vi "Read XML Parameters File_Parse Read Data_Convert sdi element.vi"(8 "error in (no error)":errorcluster, 11 "sdi":i32(ring) items=["All", "Item00", "Item01", "Item10", "Item11"]) -> (0 "error out":errorcluster, 2 "SDIValue":u8, 3 "SDI_Enabled":bool)   [LabVIEW 2019]
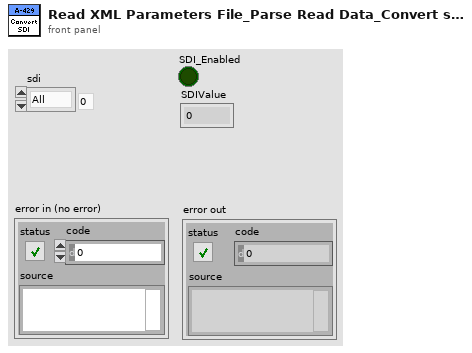
[diagram p1: front panel]
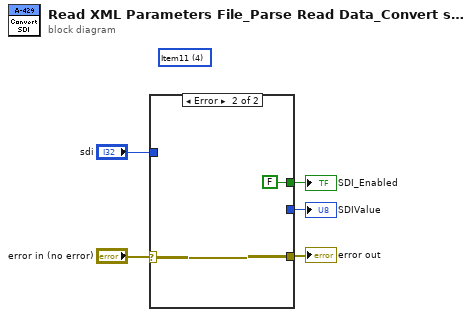
[diagram p0: block diagram]
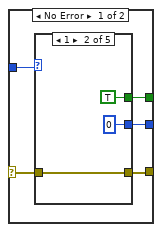
[diagram p2: hidden frame]
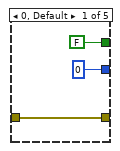
[diagram p3: hidden frame]
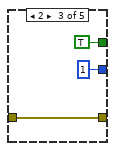
[diagram p4: hidden frame]
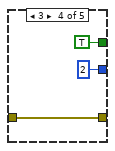
[diagram p5: hidden frame]
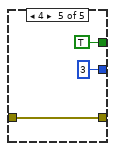
[diagram p6: hidden frame]
diagram:
  (unwired) 4 items=["All", "Item00", "Item01", "Item10", "Item11"] ("sdi")
  n1 = case shown="Error" "error in (no error)" {
    selector: "error in (no error)" -> [w9 w27]
    tunnel: [w8 w27] -> w4
    tunnel: "sdi" -> [w10 _]
    tunnel: [w7 FALSE] -> w2
    tunnel: [w6 _] -> w1
    frame No Error {
      n2 = case shown="1" w10 {
        tunnel: w9 -> [w13 w16 w19 w22 w25]
        tunnel: [w13 w16 w19 w22 w25] -> w8
        tunnel: [FALSE TRUE TRUE TRUE TRUE] -> w7
        tunnel: [u8 0 ("SDIValue") u8 0 ("SDIValue") u8 1 ("SDIValue") u8 2 ("SDIValue") u8 3 ("SDIValue")] -> w6
        frame 0, Default {
        }
        frame 1 {
        }
        frame 2 {
        }
        frame 3 {
        }
        frame 4 {
        }
      }
    }
    frame Error {
    }
  }
  "error out" <- w4
  "SDI_Enabled" <- w2
  "SDIValue" <- w1
